vi "PID r-y windup_chan.vi"(7 "PID Gains":cluster{"Kp":dbl, "Kd":dbl, "Ki":dbl}, 8 "Saturation":dbl[](array[numeric])=[-1.0, 1.0], 9 "Reverse Motor?":bool, 10 "Encoder position":dbl, 11 "Reference":dbl) -> (0 "Duty cycle":dbl, 1 "Windup (Ki Disable?)":bool, 2 "DIR":bool, 3 "Duty Cycle (Abs)":dbl)   [LabVIEW 2018]
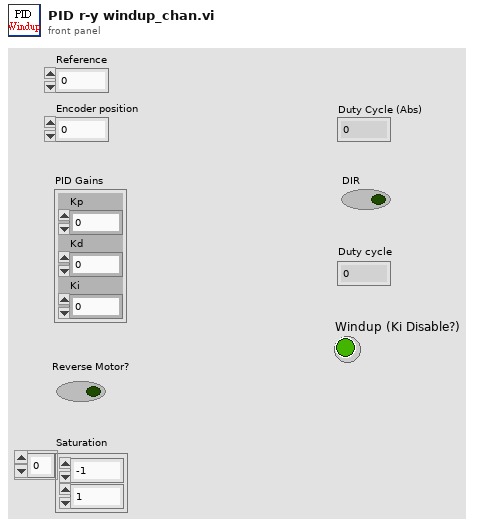
[diagram p1: front panel]
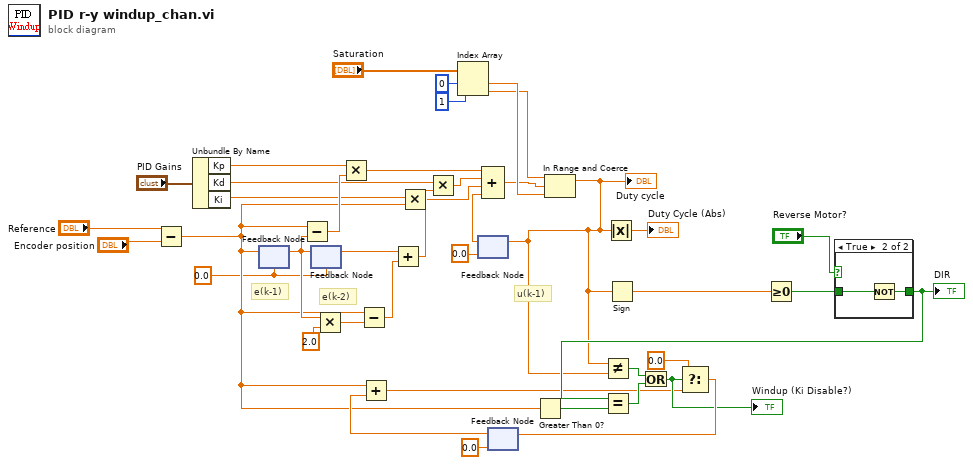
[diagram p0: block diagram]
diagram:
  w3 = 0.0
  # "e(k-2)"
  # "e(k-1)"
  # "u(k-1)"
  n1 = Subtract(x="Reference", y="Encoder position") -> (x-y=w5:dbl)
  n2 = Unbundle By Name("PID Gains") -> ("Kp"=w40:dbl, "Kd"=w16:dbl, "Ki"=w9:dbl)
  n3 = feedback #1(w3) -> (w11:dbl)
  n4 = feedback-in #1(w5) -> ()
  n5 = Subtract(x=w5, y=w11) -> (x-y=w17:dbl)
  n6 = feedback #2(w3) -> (w12:dbl)
  n7 = feedback-in #2(w11) -> ()
  n8 = Multiply(x=w11, y=2.0) -> (x*y=w14:dbl)
  n9 = Multiply(x=w40, y=w17) -> (x*y=w41:dbl)
  n10 = Subtract(x=w5, y=w14) -> (x-y=w13:dbl)
  n11 = Add(x=w12, y=w13) -> (x+y=w10:dbl)
  n12 = Multiply(x=w9, y=w5) -> (x*y=w8:dbl)
  n13 = Multiply(x=w16, y=w10) -> (x*y=w7:dbl)
  n14 = Index Array(array="Saturation", index #1=0 ("index"), index #2=1 ("index")) -> (element #1=w35:dbl, element #2=w34:dbl)
  n15 = feedback #3(0.0) -> (w6:dbl)
  n16 = Compound Arithmetic op=ADD(w41, w7, w8, w6) -> (w2:dbl)
  n17 = feedback #4(0.0 ("Ki")) -> (w21:dbl)
  n18 = Add(x=w5, y=w21) -> (x+y=w20:dbl)
  n19 = Greater Than 0?(x=w5) -> (x > 0?=w23:bool)
  n20 = In Range and Coerce(upper limit=w34, x=w2, lower limit=w35) -> (coerced(x)=w1:dbl)  [unwired: 1 out]
  "Duty cycle" <- w1
  n21 = feedback-in #3(w1) -> ()
  n22 = Not Equal?(x=w1, y=w1) -> (x != y?=w28:bool)
  n23 = Absolute Value(x=w1) -> (abs(x)=→"Duty Cycle (Abs)":dbl)
  n24 = Sign(1:w1) -> (0:w25:dbl)
  n25 = Greater Or Equal To 0?(x=w25) -> (x >= 0?=w24:bool)
  n26 = case shown="True" "Reverse Motor?" {
    tunnel: w24 -> [w42 w44]
    tunnel: [w42 w43] -> w22
    frame False {
    }
    frame True {
      n27 = Not(x=w44) -> (.not. x?=w43:bool)
    }
  }
  "DIR" <- w22
  n28 = Equal?(x=w22, y=w23) -> (x = y?=w27:bool)
  n29 = Or(x=w28, y=w27) -> (x .or. y?=w26:bool)
  "Windup (Ki Disable?)" <- w26
  n30 = Select(t=0.0, s=w26, f=w20) -> (s? t:f=w30:dbl)
  n31 = feedback-in #4(w30) -> ()
